vi "Split Message.vi"(8 "error in (no error)":errorcluster, 11 "Recipient.Message":string) -> (0 "error out":errorcluster, 2 "Message":string, 3 "Recipient":string)   [LabVIEW 2018, in "Application.lvlib" / "Message.lvclass"]
uses:
  Message.lvclass
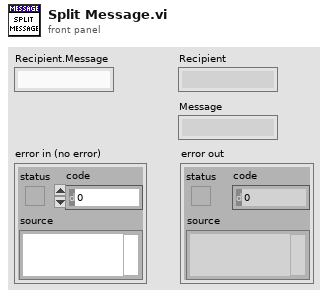
[diagram p1: front panel]
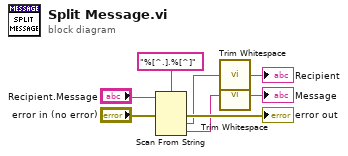
[diagram p0: block diagram]
diagram:
  n1 = Scan From String(format string="%[^.].%[^]" ("regular expression"), input string="Recipient.Message", error in="error in (no error)") -> (error out=→"error out":errorcluster, output 1=w3:string, output 2=w4:string)  [unwired: 3 in, 2 out]
  n2 = call <vilib>:"Trim Whitespace.vi"("string"=w3) -> ("trimmed string"=→"Recipient":string)  [unwired: 1 in]
  n3 = call <vilib>:"Trim Whitespace.vi"("string"=w4) -> ("trimmed string"=→"Message":string)  [unwired: 1 in]
